vi "2283_nivelesElevador.vi"(1 "Nivel 3 cajas":dbl, 2 "Nivel 2 cajas":dbl, 3 "Nivel 1 caja":dbl, 4 "Nivel cargar":dbl) -> (0 "output cluster":T1)   [LabVIEW 2014]
panel:
  in  "Niveles Elevador":T1
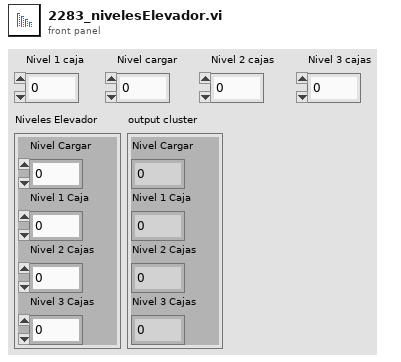
[diagram p1: front panel]
types:
  T1 = cluster{"Nivel Cargar":dbl, "Nivel 1 Caja":dbl, "Nivel 2 Cajas":dbl, "Nivel 3 Cajas":dbl}
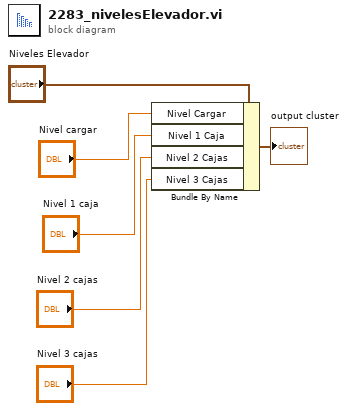
[diagram p0: block diagram]
diagram:
  n1 = Bundle By Name(cluster="Niveles Elevador", "Nivel Cargar"="Nivel cargar", "Nivel 1 Caja"="Nivel 1 caja", "Nivel 2 Cajas"="Nivel 2 cajas", "Nivel 3 Cajas"="Nivel 3 cajas") -> (→"output cluster":T1)
